vi "Hot Goal Recognition.vi"() -> (0 "Right Goal Hot?":bool, 1 "Image":T1(plugin-control), 2 "Left Goal hot?":bool)   [LabVIEW 2013]
uses:
  <vilib>/Rock Robotics/WPI/Camera/WPI_CameraSettings Read MJPG.ctl
  <vilib>/Rock Robotics/WPI/Camera/WPI_CameraImageSize.ctl
  <vilib>/vision/NI_Vision_Development_Module.lvlib
panel:
  out "ERROR":bool
  out "error out":errorcluster
  in  "Camera IP":string="10.9.0.11"
  out "Bandwidth (Mbps)":dbl
  in  "Camera Settings":T2={"fps"=30, "compression"=30, "Image Size"=enum."320x240"}
  # "do not change resolution!!!! (320x240)"
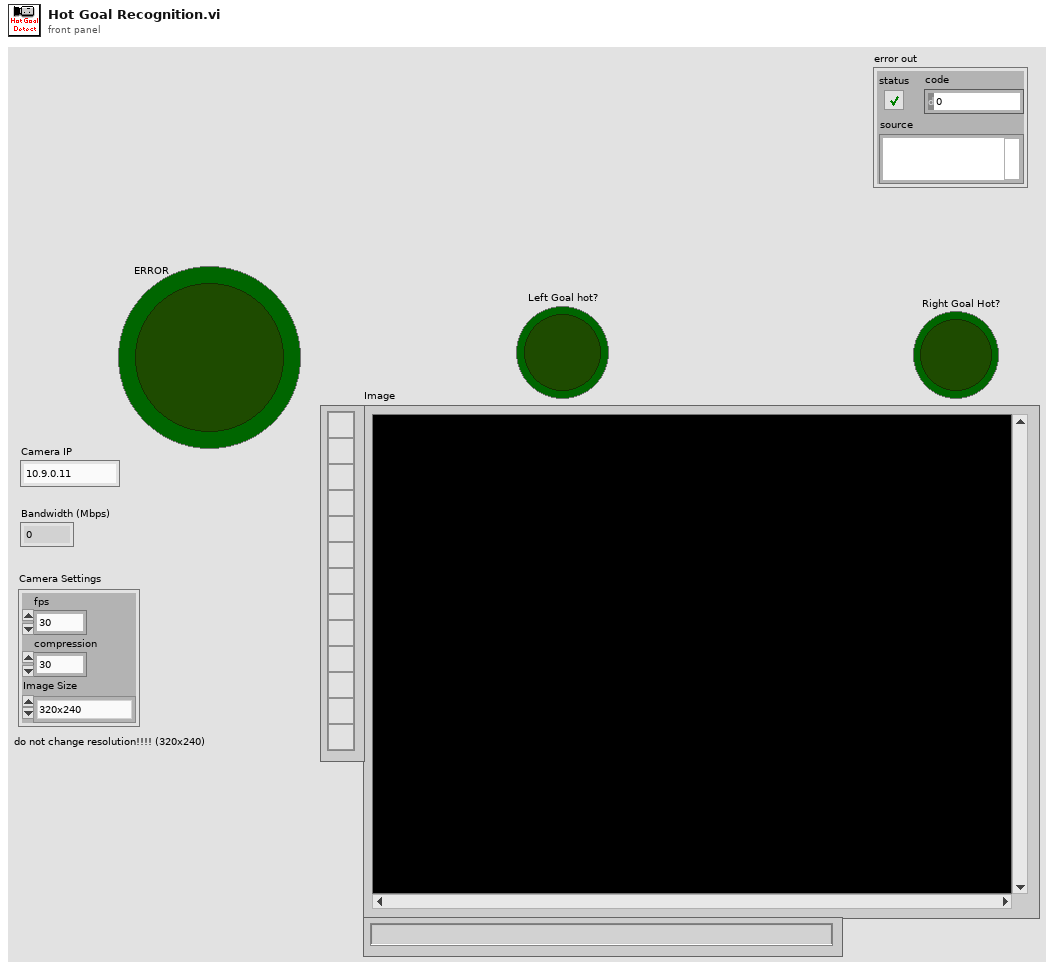
[diagram p1: front panel]
types:
  T1 = typedef "IMAQ Image.ctl" = refnum<image>
  T2 = typedef "WPI_CameraSettings Read MJPG.ctl" = cluster{"fps":i32, "compression":i32, "Image Size":T3}
  T3 = typedef "WPI_CameraImageSize.ctl" = enum16{"640x480", "320x240", "160x120"}
  T4 = typedef "Image Type" = u32
  T5 = typedef "WPI_CameraDevRef.ctl" = cluster{"Camera Address":string, "CameraStatus":errorcluster, "Acquire Image Notifier":refnum<notifier>}
  T6 = enum32{"AutoM", "Close", "Dilate", "Erode", "Gradient", "Gradient in", "Gradient out", "HitMiss", "Open", "PClose", "POpen", "Thick", "Thin"}
  T7 = typedef "Particle Parameters" = i32
  T8 = cluster{"Particle Measurements (Pixels)[0]":dbl, "Particle Measurements (Pixels)[1]":dbl}
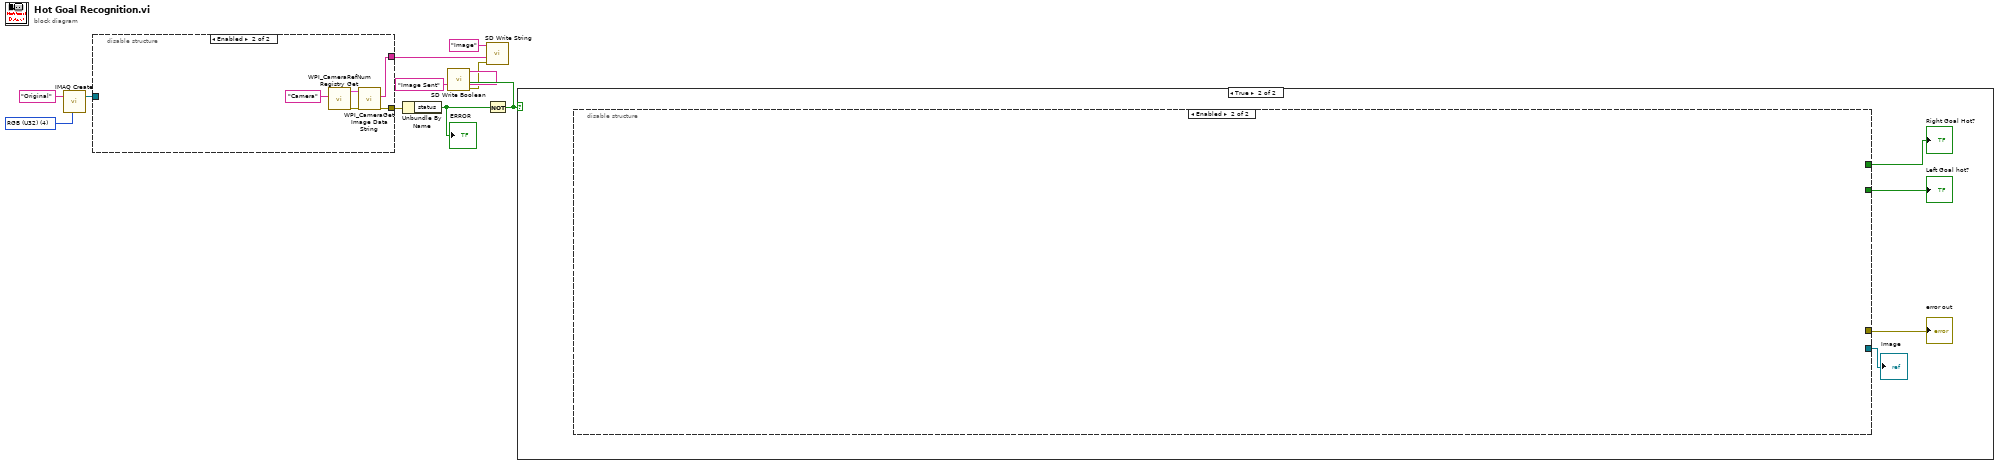
[diagram p0: block diagram]
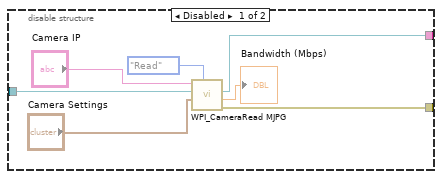
[diagram p2: hidden frame]
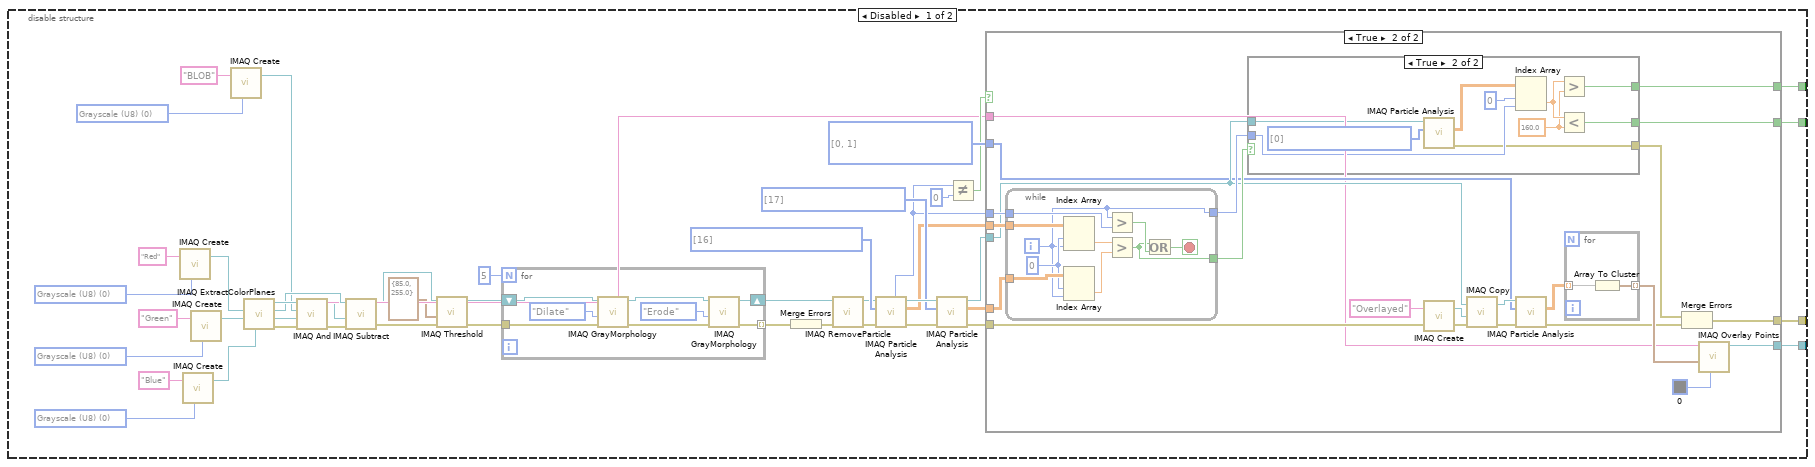
[diagram p4: hidden frame]
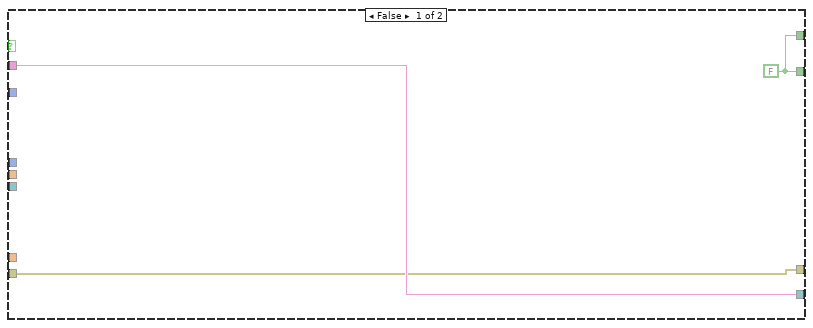
[diagram p5: hidden frame]
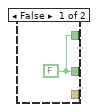
[diagram p6: hidden frame]
diagram:
  w8 = T4 4 items=["Grayscale (U8)", "Grayscale (I16)", "Grayscale (SGL)", "Complex (CSG)", "RGB (U32)", "HSL (U32)", "RGB (U64)", "Grayscale (U16)"] ("Image Type")
  n1 = call "IMAQ Create"("Image Name"="Original", "Image Type"=w8) -> ("New Image"=w6:T1)  [unwired: 3 in, 1 out]
  n2 = disable-structure shown="Enabled" {
    disable-tunnel: [w14 w19] -> w5
    disable-tunnel: [w12 w18] -> w10
    disable-tunnel: w6 -> [w11 _]
    frame Disabled {
      n3 = call <vilib>:"WPI_CameraRead MJPG.vi"("Operation"=enum16{"Read", "Reopen", "Close"}."Read", "Camera Settings"="Camera Settings", "Image"=w11, "address"="Camera IP") -> ("error out"=w12:errorcluster, "Bandwidth (Mbps)"=→"Bandwidth (Mbps)":dbl, "Image Out"=w14:T1)  [unwired: 5 in]
    }
    frame Enabled {
      n4 = call <vilib>:"WPI_CameraRefNum Registry Get.vi"("refnum name"="Camera") -> ("error out"=w22:errorcluster, "CameraDevRef"=w21:T5)  [unwired: 9 in]
      n5 = call <vilib>:"WPI_CameraGet Image Data String.vi"("error in (no error)"=w22, "CameraDevRef"=w21) -> ("error out"=w18:errorcluster, "Image Data String"=w19:string)  [unwired: 7 in, 1 out]
    }
  }
  n6 = Unbundle By Name(w10) -> ("status"=w9:bool)
  "ERROR" <- w9
  n7 = call <vilib>:"SD Write String.vi"("String"=w5, "Name"="Image") -> ("error out"=w1:errorcluster)  [unwired: 8 in, 1 out]
  n8 = Not(x=w9) -> (.not. x?=w3:bool)
  n9 = call <vilib>:"SD Write Boolean.vi"("error in"=w1, "Boolean"=w3, "Name"="Image Sent") -> ()  [unwired: 7 in, 2 out]
  n10 = case shown="True" w3 {
    frame False {
    }
    frame True {
      n11 = disable-structure shown="Enabled" {
        disable-tunnel: [w42 _] -> w26
        disable-tunnel: [w40 _] -> w25
        disable-tunnel: [w39 _] -> w24
        disable-tunnel: [w31 _] -> w23
        frame Disabled {
          w46 = T7[] [0, 1] items=["Center of Mass X", "Center of Mass Y", "First Pixel X", "First Pixel Y", "Bounding Rect Left", "Bounding Rect Top", "Bounding Rect Right", "Bounding Rect Bottom", "Max Feret Diameter Start X", "Max Feret Diameter Start Y", "Max Feret Diameter End X", "Max Feret Diameter End Y", "Max Horiz. Segment Length Left", "Max Horiz. Segment Length Right", "Max Horiz. Segment Length Row", "-", "Bounding Rect Width", "Bounding Rect Height", "Bounding Rect Diagonal", "Perimeter", "Convex Hull Perimeter", "Holes' Perimeter", "Max Feret Diameter", "Equivalent Ellipse Major Axis", "Equivalent Ellipse Minor Axis", "Equivalent Ellipse Minor Axis (Feret)", "Equivalent Rect Long Side", "Equivalent Rect Short Side", "Equivalent Rect Diagonal", "Equivalent Rect Short Side (Feret)", "Average Horiz. Segment Length", "Average Vert. Segment Length", "Hydraulic Radius", "Waddel Disk Diameter", "-", "Area", "Holes' Area", "Particle & Holes' Area", "Convex Hull Area", "Image Area", "-", "Number of Holes", "Number of Horiz. Segments", "Number of Vert. Segments", "-", "Orientation", "Max Feret Diameter Orientation", "-", "% Area/Image Area", "% Area/(Particle & Holes' Area)", "Ratio of Equivalent Ellipse Axes", "Ratio of Equivalent Rect Sides", "-", "Elongation Factor", "Compactness Factor", "Heywood Circularity Factor", "Type Factor", "-", "Sum X", "Sum Y", "Sum XX", "Sum XY", "Sum YY", "Sum XXX", "Sum XXY", "Sum XYY", "Sum YYY", "-", "Moment of Inertia XX", "Moment of Inertia XY", "Moment of Inertia YY", "Moment of Inertia XXX", "Moment of Inertia XXY", "Moment of Inertia XYY", "Moment of Inertia YYY", "Norm. Moment of Inertia XX", "Norm. Moment of Inertia XY", "Norm. Moment of Inertia YY", "Norm. Moment of Inertia XXX", "Norm. Moment of Inertia XXY", "Norm. Moment of Inertia XYY", "Norm. Moment of Inertia YYY", "Hu Moment 1", "Hu Moment 2", "Hu Moment 3", "Hu Moment 4", "Hu Moment 5", "Hu Moment 6", "Hu Moment 7"] ("Pixel Measurements")
          w58 = T4 0 items=["Grayscale (U8)", "Grayscale (I16)", "Grayscale (SGL)", "Complex (CSG)", "RGB (U32)", "HSL (U32)", "RGB (U64)", "Grayscale (U16)"] ("Image Type")
          w61 = T4 0 items=["Grayscale (U8)", "Grayscale (I16)", "Grayscale (SGL)", "Complex (CSG)", "RGB (U32)", "HSL (U32)", "RGB (U64)", "Grayscale (U16)"] ("Image Type")
          w63 = T4 0 items=["Grayscale (U8)", "Grayscale (I16)", "Grayscale (SGL)", "Complex (CSG)", "RGB (U32)", "HSL (U32)", "RGB (U64)", "Grayscale (U16)"] ("Image Type")
          w68 = T7[] [17] items=["Center of Mass X", "Center of Mass Y", "First Pixel X", "First Pixel Y", "Bounding Rect Left", "Bounding Rect Top", "Bounding Rect Right", "Bounding Rect Bottom", "Max Feret Diameter Start X", "Max Feret Diameter Start Y", "Max Feret Diameter End X", "Max Feret Diameter End Y", "Max Horiz. Segment Length Left", "Max Horiz. Segment Length Right", "Max Horiz. Segment Length Row", "-", "Bounding Rect Width", "Bounding Rect Height", "Bounding Rect Diagonal", "Perimeter", "Convex Hull Perimeter", "Holes' Perimeter", "Max Feret Diameter", "Equivalent Ellipse Major Axis", "Equivalent Ellipse Minor Axis", "Equivalent Ellipse Minor Axis (Feret)", "Equivalent Rect Long Side", "Equivalent Rect Short Side", "Equivalent Rect Diagonal", "Equivalent Rect Short Side (Feret)", "Average Horiz. Segment Length", "Average Vert. Segment Length", "Hydraulic Radius", "Waddel Disk Diameter", "-", "Area", "Holes' Area", "Particle & Holes' Area", "Convex Hull Area", "Image Area", "-", "Number of Holes", "Number of Horiz. Segments", "Number of Vert. Segments", "-", "Orientation", "Max Feret Diameter Orientation", "-", "% Area/Image Area", "% Area/(Particle & Holes' Area)", "Ratio of Equivalent Ellipse Axes", "Ratio of Equivalent Rect Sides", "-", "Elongation Factor", "Compactness Factor", "Heywood Circularity Factor", "Type Factor", "-", "Sum X", "Sum Y", "Sum XX", "Sum XY", "Sum YY", "Sum XXX", "Sum XXY", "Sum XYY", "Sum YYY", "-", "Moment of Inertia XX", "Moment of Inertia XY", "Moment of Inertia YY", "Moment of Inertia XXX", "Moment of Inertia XXY", "Moment of Inertia XYY", "Moment of Inertia YYY", "Norm. Moment of Inertia XX", "Norm. Moment of Inertia XY", "Norm. Moment of Inertia YY", "Norm. Moment of Inertia XXX", "Norm. Moment of Inertia XXY", "Norm. Moment of Inertia XYY", "Norm. Moment of Inertia YYY", "Hu Moment 1", "Hu Moment 2", "Hu Moment 3", "Hu Moment 4", "Hu Moment 5", "Hu Moment 6", "Hu Moment 7"] ("Pixel Measurements")
          w70 = T7[] [16] items=["Center of Mass X", "Center of Mass Y", "First Pixel X", "First Pixel Y", "Bounding Rect Left", "Bounding Rect Top", "Bounding Rect Right", "Bounding Rect Bottom", "Max Feret Diameter Start X", "Max Feret Diameter Start Y", "Max Feret Diameter End X", "Max Feret Diameter End Y", "Max Horiz. Segment Length Left", "Max Horiz. Segment Length Right", "Max Horiz. Segment Length Row", "-", "Bounding Rect Width", "Bounding Rect Height", "Bounding Rect Diagonal", "Perimeter", "Convex Hull Perimeter", "Holes' Perimeter", "Max Feret Diameter", "Equivalent Ellipse Major Axis", "Equivalent Ellipse Minor Axis", "Equivalent Ellipse Minor Axis (Feret)", "Equivalent Rect Long Side", "Equivalent Rect Short Side", "Equivalent Rect Diagonal", "Equivalent Rect Short Side (Feret)", "Average Horiz. Segment Length", "Average Vert. Segment Length", "Hydraulic Radius", "Waddel Disk Diameter", "-", "Area", "Holes' Area", "Particle & Holes' Area", "Convex Hull Area", "Image Area", "-", "Number of Holes", "Number of Horiz. Segments", "Number of Vert. Segments", "-", "Orientation", "Max Feret Diameter Orientation", "-", "% Area/Image Area", "% Area/(Particle & Holes' Area)", "Ratio of Equivalent Ellipse Axes", "Ratio of Equivalent Rect Sides", "-", "Elongation Factor", "Compactness Factor", "Heywood Circularity Factor", "Type Factor", "-", "Sum X", "Sum Y", "Sum XX", "Sum XY", "Sum YY", "Sum XXX", "Sum XXY", "Sum XYY", "Sum YYY", "-", "Moment of Inertia XX", "Moment of Inertia XY", "Moment of Inertia YY", "Moment of Inertia XXX", "Moment of Inertia XXY", "Moment of Inertia XYY", "Moment of Inertia YYY", "Norm. Moment of Inertia XX", "Norm. Moment of Inertia XY", "Norm. Moment of Inertia YY", "Norm. Moment of Inertia XXX", "Norm. Moment of Inertia XXY", "Norm. Moment of Inertia XYY", "Norm. Moment of Inertia YYY", "Hu Moment 1", "Hu Moment 2", "Hu Moment 3", "Hu Moment 4", "Hu Moment 5", "Hu Moment 6", "Hu Moment 7"] ("Pixel Measurements")
          w71 = T4 0 items=["Grayscale (U8)", "Grayscale (I16)", "Grayscale (SGL)", "Complex (CSG)", "RGB (U32)", "HSL (U32)", "RGB (U64)", "Grayscale (U16)"] ("Image Type")
          n12 = call "IMAQ Create"("Image Name"="Red", "Image Type"=w63) -> ("New Image"=w64:T1)  [unwired: 3 in, 1 out]
          n13 = call "IMAQ Create"("Image Name"="Blue", "Image Type"=w58) -> ("New Image"=w57:T1)  [unwired: 3 in, 1 out]
          n14 = call "IMAQ Create"("Image Name"="Green", "Image Type"=w61) -> ("New Image"=w60:T1)  [unwired: 3 in, 1 out]
          n15 = call "IMAQ Create"("Image Name"="BLOB", "Image Type"=w71) -> ("New Image"=w28:T1)  [unwired: 3 in, 1 out]
          n16 = call "IMAQ ExtractColorPlanes"("Blue or Luma or Val or Inten Plane"=w57, "Green or Sat Plane"=w60, "Red or Hue Plane"=w64, "Image Src"=w41) -> ("error out"=w38:errorcluster, "Blue or Luma or Val or Inten Plane out"=w55:T1, "Green or Sat Plane out"=w54:T1, "Red or Hue Plane out"=w56:T1)  [unwired: 4 in]
          n17 = call "IMAQ And"("error in (no error)"=w38, "Image Src B"=w55, "Image Dst"=w28, "Image Src A"=w56) -> ("error out"=w35:errorcluster, "Image Dst Out"=w27:T1)  [unwired: 6 in]
          n18 = call "IMAQ Subtract"("Image Src A"=w54, "Image Src B"=w27, "error in (no error)"=w35) -> ("Image Dst Out"=w36:T1, "error out"=w34:errorcluster)  [unwired: 4 in]
          n19 = call "IMAQ Threshold"("error in (no error)"=w34, "Range"=cluster{"Lower value":sgl, "Upper value":sgl} {"Lower value"=85.0, "Upper value"=255.0}, "Image Src"=w36) -> ("error out"=w33:errorcluster, "Image Dst Out"=w37:T1)  [unwired: 7 in]
          n20 = for {
            N: 5 -> [_]
            shift-right: [w76] -> w29
            shift-left: w37 -> [w77]
            tunnel: w33 -> [w75]
            tunnel: [w73] -> w52 mode=indexing
            n21 = call "IMAQ GrayMorphology"("error in (no error)"=w75, "Operation"=T6."Dilate", "Image Src"=w77) -> ("error out"=w74:errorcluster, "Image Dst Out"=w78:T1)  [unwired: 7 in]
            n22 = call "IMAQ GrayMorphology"("error in (no error)"=w74, "Operation"=T6."Erode", "Image Src"=w78) -> ("error out"=w73:errorcluster, "Image Dst Out"=w76:T1)  [unwired: 7 in]
          }
          n23 = Merge Errors(w52) -> (w30:errorcluster)
          n24 = call "IMAQ RemoveParticle"("error in (no error)"=w30, "Image Src"=w29) -> ("error out"=w49:errorcluster, "Image Dst Out"=w50:T1)  [unwired: 8 in]
          n25 = call "IMAQ Particle Analysis"("error in (no error)"=w49, "Pixel Measurements"=w70, "Image"=w50) -> ("error out"=w51:errorcluster, "Particle Measurements (Pixels)"=w67:dbl[][], "Image Out (duplicate)"=w69:T1, "Number of Particles"=w45:i32)  [unwired: 3 in, 2 out]
          n26 = call "IMAQ Particle Analysis"("error in (no error)"=w51, "Pixel Measurements"=w68, "Image"=w69) -> ("error out"=w47:errorcluster, "Particle Measurements (Pixels)"=w66:dbl[][], "Image Out (duplicate)"=w48:T1)  [unwired: 3 in, 3 out]
          n27 = Not Equal?(x=w45, y=0) -> (x != y?=w43:bool)
          n28 = case shown="True" w43 {
            tunnel: w67 -> [_ w106]
            tunnel: w66 -> [_ w105]
            tunnel: w45 -> [_ w104]
            tunnel: w48 -> [_ w99]
            tunnel: w47 -> [w81 w98]
            tunnel: w46 -> [_ w94]
            tunnel: [w83 w90] -> w42
            tunnel: [w83 w89] -> w41
            tunnel: [w82 w88] -> w40
            tunnel: [w82 w87] -> w39
            tunnel: [w81 w84] -> w31
            frame False {
              w82 = FALSE
            }
            frame True {
              n29 = while {
                tunnel: w106 -> [w128]
                tunnel: w105 -> [w129]
                tunnel: w104 -> [w122]
                tunnel: [w121] -> w102
                tunnel: [w120] -> w103
                i -> [w120]
                stop <- w123 stop-if-true
                w127 = 0 ("disabled index (row)")
                n30 = Index Array(array=w128, index (row)=w127, index (col)=w120) -> (element=w125:dbl)
                n31 = Index Array(array=w129, index (row)=w127, index (col)=w120) -> (element=w126:dbl)
                n32 = Greater?(x=w120, y=w122) -> (0:w124:bool)
                n33 = Greater?(x=w125, y=w126) -> (0:w121:bool)
                n34 = Or(x=w121, y=w124) -> (x .or. y?=w123:bool)
              }
              n35 = case shown="True" w102 {
                tunnel: w103 -> [_ w115]
                tunnel: w99 -> [_ w118]
                tunnel: [_ w114] -> w85
                tunnel: [w109 w111] -> w88
                tunnel: [w109 w110] -> w87
                frame False {
                  w109 = FALSE
                }
                frame True {
                  w112 = 160.0 ("y")
                  w119 = T7[] [0] items=["Center of Mass X", "Center of Mass Y", "First Pixel X", "First Pixel Y", "Bounding Rect Left", "Bounding Rect Top", "Bounding Rect Right", "Bounding Rect Bottom", "Max Feret Diameter Start X", "Max Feret Diameter Start Y", "Max Feret Diameter End X", "Max Feret Diameter End Y", "Max Horiz. Segment Length Left", "Max Horiz. Segment Length Right", "Max Horiz. Segment Length Row", "-", "Bounding Rect Width", "Bounding Rect Height", "Bounding Rect Diagonal", "Perimeter", "Convex Hull Perimeter", "Holes' Perimeter", "Max Feret Diameter", "Equivalent Ellipse Major Axis", "Equivalent Ellipse Minor Axis", "Equivalent Ellipse Minor Axis (Feret)", "Equivalent Rect Long Side", "Equivalent Rect Short Side", "Equivalent Rect Diagonal", "Equivalent Rect Short Side (Feret)", "Average Horiz. Segment Length", "Average Vert. Segment Length", "Hydraulic Radius", "Waddel Disk Diameter", "-", "Area", "Holes' Area", "Particle & Holes' Area", "Convex Hull Area", "Image Area", "-", "Number of Holes", "Number of Horiz. Segments", "Number of Vert. Segments", "-", "Orientation", "Max Feret Diameter Orientation", "-", "% Area/Image Area", "% Area/(Particle & Holes' Area)", "Ratio of Equivalent Ellipse Axes", "Ratio of Equivalent Rect Sides", "-", "Elongation Factor", "Compactness Factor", "Heywood Circularity Factor", "Type Factor", "-", "Sum X", "Sum Y", "Sum XX", "Sum XY", "Sum YY", "Sum XXX", "Sum XXY", "Sum XYY", "Sum YYY", "-", "Moment of Inertia XX", "Moment of Inertia XY", "Moment of Inertia YY", "Moment of Inertia XXX", "Moment of Inertia XXY", "Moment of Inertia XYY", "Moment of Inertia YYY", "Norm. Moment of Inertia XX", "Norm. Moment of Inertia XY", "Norm. Moment of Inertia YY", "Norm. Moment of Inertia XXX", "Norm. Moment of Inertia XXY", "Norm. Moment of Inertia XYY", "Norm. Moment of Inertia YYY", "Hu Moment 1", "Hu Moment 2", "Hu Moment 3", "Hu Moment 4", "Hu Moment 5", "Hu Moment 6", "Hu Moment 7"] ("Pixel Measurements")
                  n36 = call "IMAQ Particle Analysis"("Pixel Measurements"=w119, "Image"=w118) -> ("error out"=w114:errorcluster, "Particle Measurements (Pixels)"=w117:dbl[][])  [unwired: 4 in, 4 out]
                  n37 = Index Array(array=w117, index (row)=0, index (col)=w115) -> (element=w113:dbl)
                  n38 = Greater?(x=w113, y=w112) -> (0:w111:bool)
                  n39 = Less?(x=w113, y=w112) -> (x < y?=w110:bool)
                }
              }
              n40 = call "IMAQ Create"("Image Name"="Overlayed", "error in (no error)"=w98) -> ("New Image"=w100:T1, "error out"=w97:errorcluster)  [unwired: 3 in]
              n41 = call "IMAQ Copy"("error in (no error)"=w97, "Image Dst"=w100, "Image Src"=w99) -> ("error out"=w96:errorcluster, "Image Dst Out"=w95:T1)  [unwired: 3 in]
              n42 = call "IMAQ Particle Analysis"("error in (no error)"=w96, "Pixel Measurements"=w94, "Image"=w95) -> ("error out"=w86:errorcluster, "Particle Measurements (Pixels)"=w91:dbl[][])  [unwired: 3 in, 4 out]
              n43 = for {
                tunnel: w91 -> [w108] mode=indexing
                tunnel: [w107] -> w92 mode=indexing
                n44 = Array To Cluster(array=w108) -> (cluster=w107:T8)
              }
              n45 = Merge Errors(w85, w86) -> (w84:errorcluster)
              n46 = call "IMAQ Overlay Points"("Color"=u32 0, "Array of Points"=w92, "Image"=w89) -> ("Image Out"=w90:T1)  [unwired: 7 in, 1 out]
            }
          }
        }
        frame Enabled {
        }
      }
      "error out" <- w23
      "Image" <- w26
      "Right Goal Hot?" <- w25
      "Left Goal hot?" <- w24
    }
  }
